vi "Handle Events.vi"(8 "error in (no error)":errorcluster, 11 "VIEventHandler":refnum<class "VIEventHandler.lvclass">) -> ()   [LabVIEW 2020, in "ActorEvents.lvlib" / "VIEventHandler.lvclass"]
doc: "处理事件"
uses:
  VIEventHandler.lvclass
  VIEventHandler.lvclass/VIEventHandler.ctl
  IEventHandler/IEventHandler.lvclass/IEventHandler.ctl
  <vilib>/ActorFramework/Message Enqueuer/Message Enqueuer.lvclass/Message Enqueuer.ctl
  <vilib>/event_ctls.llb/lveventtype.ctl
  IEventAggregator Messages/MenuSelectionMsg/MenuSelectionMsg.lvclass/MenuSelectionMsg.ctl
  IEventAggregator Messages/EventDataMessage/EventDataMessage.lvclass/EventDataMessage.ctl
  IEventAggregator Messages/VIKeyDownMsg/VIKeyDownMsg.lvclass/VIKeyDownMsg.ctl
  IEventAggregator Messages/VIKeyDownMsg/Accessors/Read Char.vi
  IEventAggregator Messages/VIKeyDownMsg/Accessors/Read VKey.vi
  IEventAggregator Messages/VIKeyDownMsg/Accessors/Read Mods.vi
  IEventAggregator Messages/VIKeyDownMsg/Accessors/Read PlatMods.vi
  IEventAggregator Messages/VIKeyDownMsg/Accessors/Read FocusObj.vi
  IEventAggregator Messages/EventDataMessage/Read Discarded.vi
  IEventHandler/Accessors/Read Timeout [ms].vi
  IEventHandler/Accessors/Read Event Filter.vi
  IEventHandler/Accessors/Read EventAggregator Enqueuer.vi
  IEventHandler/Accessors/Read Timeout Message.vi
  IEventHandler/Accessors/Read Timeout Message Priority.vi
  IEventAggregator Messages/EventDataMessage/Send Event Data Message.vi
  <vilib>/Utility/error.llb/Clear Errors.vi
  IEventAggregator Messages/MenuSelectionMsg/MenuSelectionMsg.lvclass
  IEventAggregator Messages/EventDataMessage/EventDataMessage.lvclass
  C:/Program Files/National Instruments/LabVIEW 2020/vi.lib/ActorFramework/Message/Message.lvclass
  IEventAggregator Messages/VIKeyDownMsg/VIKeyDownMsg.lvclass
  IEventAggregator Messages/PanelCloseMsg/PanelCloseMsg.lvclass
  <vilib>/ActorFramework/Message Priority Queue/Priority Enqueue.vi
  IEventFilter/IEventFilter.lvclass
  <vilib>/ActorFramework/Message Enqueuer/Message Enqueuer.lvclass
  <vilib>/ActorFramework/Message/Message.lvclass
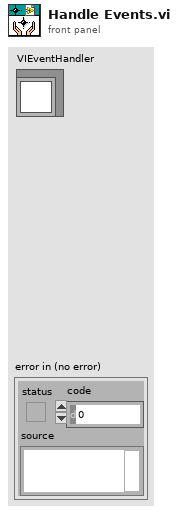
[diagram p1: front panel]
types:
  T1 = typedef "ActorEvents.lvlib/IEventFilter.lvclass/EventFilter Reference.ctl" = refnum<data-value>
  T2 = typedef "Actor Framework.lvlib/Message Enqueuer.lvclass/Message Priority.ctl" = enum16{"Low", "Normal", "High"}
  T3 = typedef "lveventtype.ctl" = enum32{"Null", "Timeout", "Annotation Menu Selection", "Annotation Menu Selection?", "App Instance Close", "App Instance Close?", "Autoscale Range Change", "Bookmark Info Change", "Cell Edit", "Cell Edit?", "Cursor Grab", "Cursor Grab?", "Cursor Menu Selection", "Cursor Menu Selection?", "Cursor Move", "Cursor Release", "Data Change", "Direction Change", "Display State Change", "Drag Ended", "Drag Enter", "Drag Leave", "Drag Over", "Drag Source Update", "Drag Starting", "Drag Starting?", "Drop", "Exec State Change", "Key Down", "Key Down?", "Key Repeat", "Key Repeat?", "Key Up", "Listbox Double Click", "Menu Activation?", "Menu Selection (App)", "Menu Selection? (App)", "Menu Selection (User)", "Mouse Down", "Mouse Down?", "Mouse Enter", "Mouse Leave", "Mouse Move", "Mouse Up", "Mouse Wheel", "NI Security User Change (App)", "Pane Size", "Panel Close", "Panel Close?", "Panel Resize", "Plot Attribute Change", "Scale Range Change", "Shortcut Menu Activation?", "Shortcut Menu Selection (App)", "Shortcut Menu Selection? (App)", "Shortcut Menu Selection (User)", "Tree Double Click", "Tree Drag", "Tree Drag?", "Tree Drop", "Tree Drop?", "Tree Item Close", "Tree Item Close?", "Tree Item Open", "Tree Item Open?", "User Event", "Value Change"}
  T4 = typedef "eventvkey.ctl" = enum16{"ASCII", "Enter", "Return", "Shift", "Ctrl", "Alt", "Cmd", "Opt", "Caps", "NumLock", "Clear", "Break", "Up", "Down", "Left", "Right", "Insert", "Delete", "Home", "End", "PageUp", "PageDown", "Escape", "Help", "Pause", "ScrollLock", "F1", "F2", "F3", "F4", "F5", "F6", "F7", "F8", "F9", "F10", "F11", "F12", "F13", "F14", "F15", "F16", "F17", "F18", "F19", "F20", "F21", "F22", "F23", "F24", "Play", "VolumeUp", "VolumeDown", "Mute", "Two Byte Char"}
  T5 = cluster{"Shift":bool, "Ctrl":bool, "Alt":bool, "Cmd":bool, "Opt":bool}
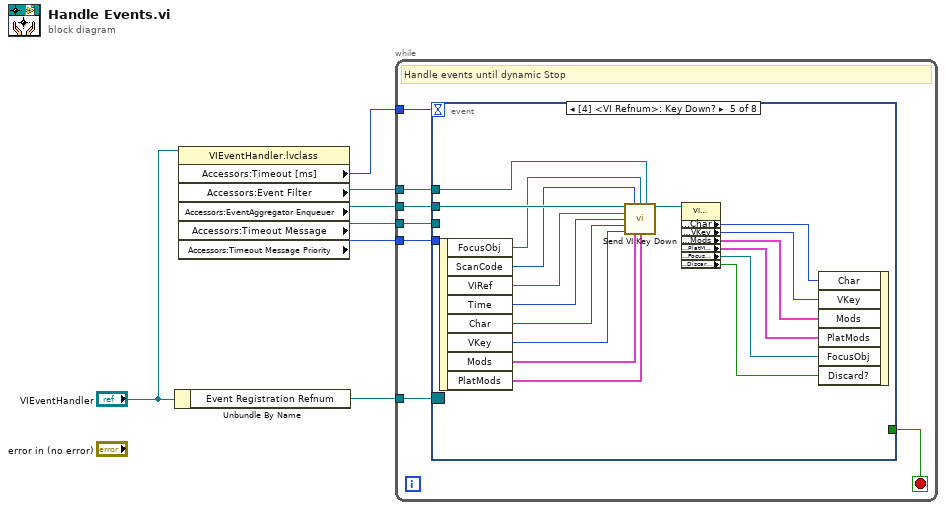
[diagram p0: block diagram]
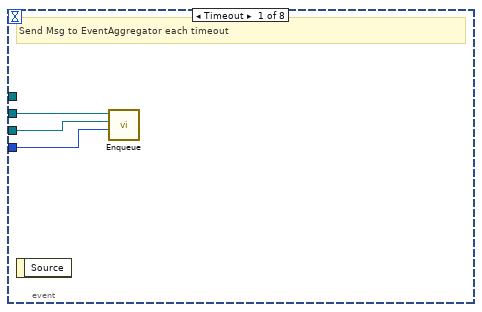
[diagram p2: hidden frame]
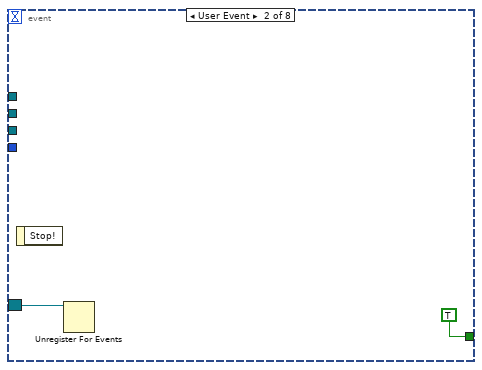
[diagram p3: hidden frame]
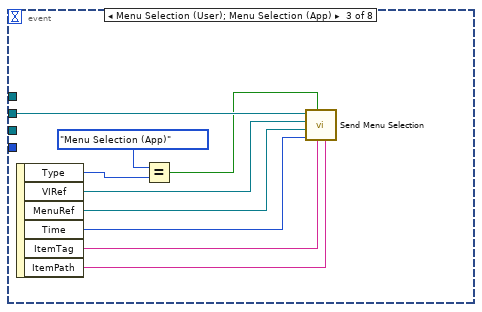
[diagram p4: hidden frame]
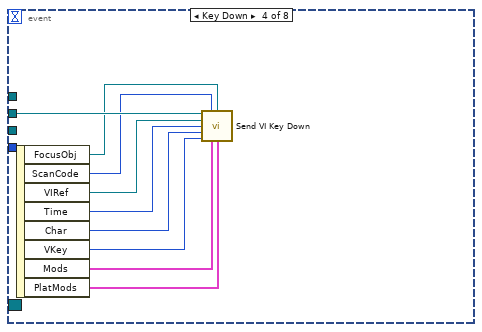
[diagram p5: hidden frame]
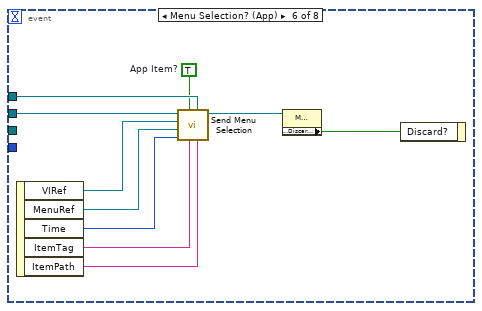
[diagram p6: hidden frame]
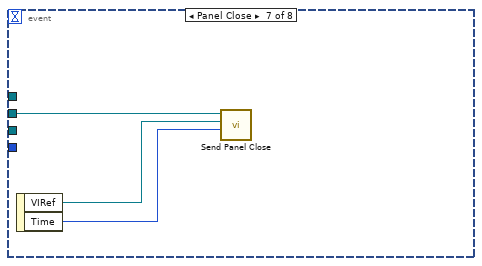
[diagram p7: hidden frame]
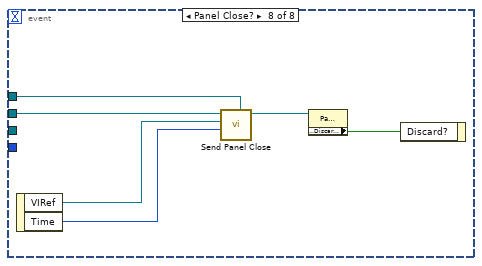
[diagram p8: hidden frame]
diagram:
  n1 = Unbundle By Name("VIEventHandler") -> ("Event Registration Refnum"=w7:refnum<event-registration>)
  n2 = property class="VIEventHandler.lvclass"(reference="VIEventHandler") -> ("Accessors:Timeout [ms]"=w5:i32, "Accessors:Event Filter"=w1:T1, "Accessors:EventAggregator Enqueuer"=w4:refnum<class "Message Enqueuer.lvclass">, "Accessors:Timeout Message"=w3:refnum<class "Message.lvclass">, "Accessors:Timeout Message Priority"=w2:T2)  [unwired: 1 in, 2 out]
  n3 = while {
    tunnel: w7 -> [w14]
    tunnel: w4 -> [w12]
    tunnel: w3 -> [w11]
    tunnel: w2 -> [w10]
    tunnel: w5 -> [w9]
    tunnel: w1 -> [w8]
    stop <- w13 stop-if-true
    # "Handle events until dynamic Stop"
    n4 = event shown="[4] <VI Refnum>: Key Down?" {
      selector: w14 -> [_ w19 _ _ _ _ _ _]
      dyn-events: _ -> [_ _ _ _ _ _ _ _]
      timeout: w9 -> [_ _ _ _ _ _ _ _]
      tunnel: [_ TRUE ("Stop!") _ _ _ _ _ _] -> w13
      tunnel: w12 -> [w17 _ w28 w37 w53 w64 w67 w73]
      tunnel: w11 -> [w16 _ _ _ _ _ _ _]
      tunnel: w10 -> [w15 _ _ _ _ _ _ _]
      tunnel: w8 -> [_ _ _ _ w54 w58 _ w69]
      event Timeout {
        # "Send Msg to EventAggregator each timeout"
        n5 = event-data() -> ()  [unwired: 1 in, 1 out]
        n6 = call <vilib>:"Enqueue.vi"("Message Priority (Normal)"=w15, "Message"=w16, "Message Enqueuer in"=w17) -> ()  [unwired: 7 in, 2 out]
      }
      event User Event {
        n7 = event-data() -> ()  [unwired: 1 in, 1 out]
        n8 = Unregister For Events(event registration refnum=w19) -> ()  [unwired: 1 in, 1 out]
      }
      event Menu Selection (User); Menu Selection (App) {
        n9 = event-data() -> ("Type"=w22:T3, "VIRef"=w23:refnum<vi>, "MenuRef"=w24:refnum<k9>, "Time"=w25:u32, "ItemTag"=w27:string, "ItemPath"=w26:string)  [unwired: 1 in]
        n10 = Equal?(x=lveventtype."Menu Selection (App)", y=w22) -> (x = y?=w21:bool)
        n11 = call "Send Menu Selection.vi"("Item Path"=w26, "Item Tag"=w27, "App Item?"=w21, "Time"=w25, "MenuRef"=w24, "VI Refnum"=w23, "Message Enqueuer in"=w28) -> ()  [unwired: 3 in, 2 out]
      }
      event Key Down {
        n12 = event-data() -> ("FocusObj"=w36:refnum<vi>, "ScanCode"=w35:i16, "VIRef"=w34:refnum<vi>, "Time"=w33:u32, "Char"=w32:i16, "VKey"=w31:T4, "Mods"=w30:cluster{"Num Pad":bool, "Menu Key":bool}, "PlatMods"=w29:T5)  [unwired: 1 in]
        n13 = call "Send VI Key Down.vi"("Message Enqueuer in"=w37, "ScanCode"=w35, "FocusObj"=w36, "VIRef"=w34, "Time"=w33, "Char"=w32, "VKey"=w31, "Mods"=w30, "PlatMods"=w29) -> ()  [unwired: 5 in, 2 out]
      }
      event Key Down? {
        n14 = event-data() -> ("FocusObj"=w52:refnum<vi>, "ScanCode"=w51:i16, "VIRef"=w50:refnum<vi>, "Time"=w49:u32, "Char"=w48:i16, "VKey"=w47:T4, "Mods"=w46:cluster{"Num Pad":bool, "Menu Key":bool}, "PlatMods"=w45:T5)  [unwired: 1 in]
        n15 = call "Send VI Key Down.vi"("Message Enqueuer in"=w53, "ScanCode"=w51, "FocusObj"=w52, "EventFilter Reference"=w54, "VIRef"=w50, "Time"=w49, "Char"=w48, "VKey"=w47, "Mods"=w46, "PlatMods"=w45) -> ("VIKeyDownMsg out"=w44:refnum<class "VIKeyDownMsg.lvclass">)  [unwired: 4 in, 1 out]
        n16 = property class="VIKeyDownMsg.lvclass"(reference=w44) -> ("Accessors:Char"=w43:i16, "Accessors:VKey"=w42:T4, "Accessors:Mods"=w41:cluster{"Double Click":bool, "Menu Key":bool}, "Accessors:PlatMods"=w40:T5, "Accessors:FocusObj"=w39:refnum<vi>, "Accessors:Discarded?"=w38:bool)  [unwired: 1 in, 2 out]
        n17 = event-data("Char"=w43, "VKey"=w42, "Mods"=w41, "PlatMods"=w40, "FocusObj"=w39, "Discard?"=w38) -> ()  [unwired: 1 in, 1 out]
      }
      event Menu Selection? (App) {
        w57 = TRUE  # App Item?
        n18 = event-data() -> ("VIRef"=w59:refnum<vi>, "MenuRef"=w60:refnum<k9>, "Time"=w61:u32, "ItemTag"=w63:string, "ItemPath"=w62:string)  [unwired: 1 in]
        n19 = call "Send Menu Selection.vi"("Item Path"=w62, "EventFilter Reference"=w58, "Item Tag"=w63, "App Item?"=w57, "Time"=w61, "MenuRef"=w60, "VI Refnum"=w59, "Message Enqueuer in"=w64) -> ("Filtered EventDataMessage"=w56:refnum<class "MenuSelectionMsg.lvclass">)  [unwired: 2 in, 1 out]
        n20 = property class="MenuSelectionMsg.lvclass"(reference=w56) -> ("Accessors:Discarded?"=w55:bool)  [unwired: 1 in, 2 out]
        n21 = event-data("Discard?"=w55) -> ()  [unwired: 1 in, 1 out]
      }
      event Panel Close {
        n22 = event-data() -> ("VIRef"=w66:refnum<vi>, "Time"=w65:u32)  [unwired: 1 in]
        n23 = call "Send Panel Close.vi"("Time"=w65, "VI Refnum"=w66, "Message Enqueuer in"=w67) -> ()  [unwired: 7 in, 2 out]
      }
      event Panel Close? {
        n24 = event-data() -> ("VIRef"=w72:refnum<vi>, "Time"=w71:u32)  [unwired: 1 in]
        n25 = call "Send Panel Close.vi"("EventFilter Reference"=w69, "Time"=w71, "VI Refnum"=w72, "Message Enqueuer in"=w73) -> ("Filtered EventDataMessage"=w70:refnum<class "PanelCloseMsg.lvclass">)  [unwired: 6 in, 1 out]
        n26 = property class="PanelCloseMsg.lvclass"(reference=w70) -> ("Accessors:Discarded?"=w68:bool)  [unwired: 1 in, 2 out]
        n27 = event-data("Discard?"=w68) -> ()  [unwired: 1 in, 1 out]
      }
    }
  }
